vi "Server.vi"() -> ()   [LabVIEW 2017]
panel:
  in  "Num":i32=100 caption="Num Elements to Generate"
  in  "Generate":bool
  in  "stop":bool
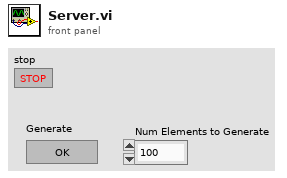
[diagram p1: front panel]
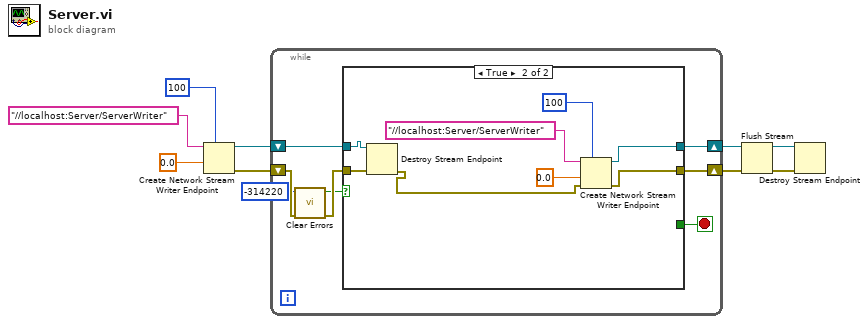
[diagram p0: block diagram]
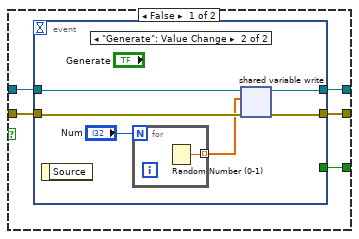
[diagram p2: hidden frame]
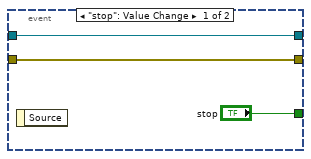
[diagram p3: hidden frame]
diagram:
  n1 = Create Network Stream Writer Endpoint(7:100 ("writer buffer size"), 9:0.0, 11:"//localhost:Server/ServerWriter" ("writer name")) -> (0:w8:errorcluster, 3:w9:refnum<k21>)  [unwired: 4 in]
  n2 = while {
    shift-right: [w16] -> w6
    shift-left: w9 -> [w15]
    shift-right: [w14] -> w7
    shift-left: w8 -> [w13]
    stop <- w17 stop-if-true
    n3 = call <vilib>:"Clear Errors.vi"("error in (no error)"=w13, "specific error code to clear (0: all)"=-314220) -> ("error out"=w12:errorcluster, "specific error cleared?"=w10:bool)  [unwired: 4 in]
    n4 = case shown="True" w10 {
      tunnel: [w22 _] -> w17
      tunnel: [w21 w35] -> w16
      tunnel: w15 -> [w20 w40]
      tunnel: w12 -> [w19 w39]
      tunnel: [w18 w34] -> w14
      frame False {
        n5 = event shown="[1] \"Generate\": Value Change" {
          selector: _ -> [_ _]
          dyn-events: _ -> [_ _]
          timeout: _ -> [_ _]
          tunnel: ["stop" _] -> w22
          tunnel: [w24 w28] -> w21
          tunnel: w20 -> [w24 w30]
          tunnel: w19 -> [w23 w29]
          tunnel: [w23 w27] -> w18
          event "stop": Value Change {
            n6 = event-data() -> ()  [unwired: 1 in, 1 out]
          }
          event "Generate": Value Change {
            n7 = event-data() -> ()  [unwired: 1 in, 1 out]
            n8 = for {
              N: "Num" -> [_]
              tunnel: [w32] -> w26 mode=indexing
              n9 = Random Number (0-1)() -> (number: 0 to 1=w32:dbl)
            }
            n10 = shared-variable-write(w30, w29, w26) -> (w28:refnum<k21>, w27:errorcluster)  [unwired: 1 in, 1 out]
          }
        }
      }
      frame True {
        n11 = Destroy Stream Endpoint(8:w39, 11:w40) -> (0:w33:errorcluster)
        n12 = Create Network Stream Writer Endpoint(7:100 ("writer buffer size"), 8:w33, 9:0.0, 11:"//localhost:Server/ServerWriter" ("writer name")) -> (0:w34:errorcluster, 3:w35:refnum<k21>)  [unwired: 3 in]
      }
    }
  }
  n13 = Flush Stream(8:w7, 11:w6) -> (0:w5:errorcluster, 3:w4:refnum<k21>)  [unwired: 2 in, 1 out]
  n14 = Destroy Stream Endpoint(8:w5, 11:w4) -> ()  [unwired: 1 out]
